vi "Skyline Send Waveform File.vi"(8 "error in":errorcluster, 9 "properties":cluster{"Key":string, "Value":string}[](array[cluster]) caption="properties (null)", 11 "data in":waveform(dbl)[](array[waveform])) -> (0 "error out":errorcluster, 2 "size in bytes":i32, 3 "data out":waveform(dbl)[](array[waveform]))   [LabVIEW 2017, in "Logger.lvclass"]
uses:
  logger/Logger.lvclass
  <vilib>/Skyline/File/File/Send Buffer.vi
  <vilib>/Skyline/File/File/NI Skyline File.lvclass
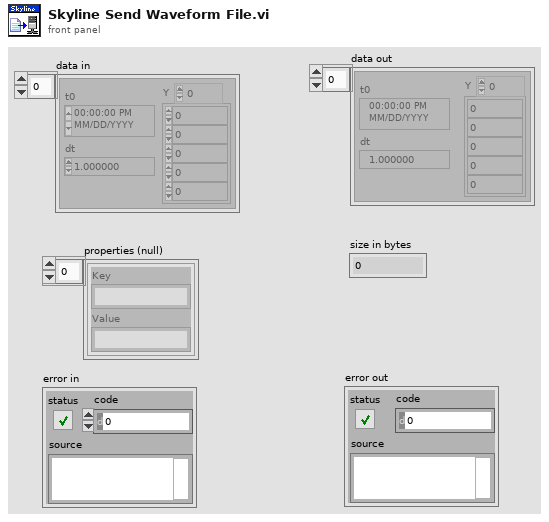
[diagram p1: front panel]
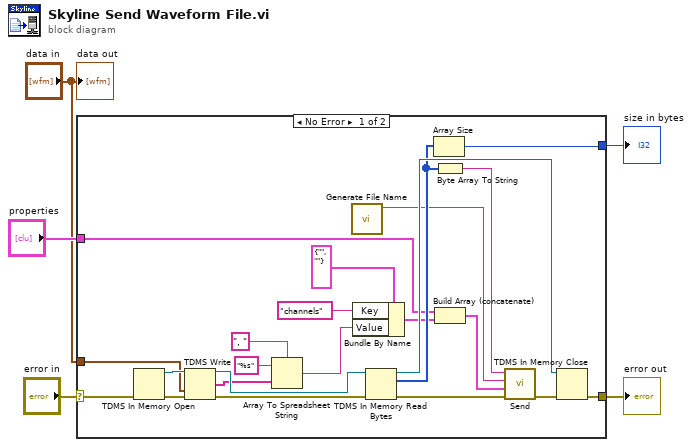
[diagram p0: block diagram]
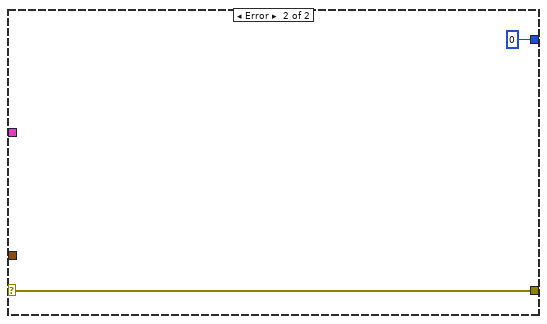
[diagram p2: hidden frame]
diagram:
  n1 = case shown="No Error" "error in" {
    selector: "error in" -> [w22 w30]
    tunnel: [w24 w30] -> w5
    tunnel: "properties" -> [w12 _]
    tunnel: "data in" -> [w27 _]
    tunnel: [w20 0] -> w1
    frame No Error {
      n2 = TDMS In Memory Open(8:w22) -> (0:w23:errorcluster, 3:w28:refnum<k34>)  [unwired: 1 in]
      n3 = TDMS Write(0:w28, 9:w27, 11:w23) -> (4:w19:refnum<k34>, 8:w17:string[], 15:w26:errorcluster)  [unwired: 3 in, 1 out]
      n4 = Array To Spreadsheet String(delimiter (Tab)=", ", array=w17, 3:"%s" ("format string")) -> (spreadsheet string=w13:string)
      n5 = call "Generate File Name.vi"() -> ("file name"=w10:string)  [unwired: 11 in]
      n6 = Bundle By Name(cluster=cluster{"Key":string, "Value":string} {"Key"="", "Value"=""} ("Property"), "Key"="channels", "Value"=w13) -> (w11:cluster{"Key":string, "Value":string})
      n7 = TDMS In Memory Read Bytes(8:w26, 11:w19) -> (0:w7:errorcluster, 2:w21:u8[], 3:w25:refnum<k34>)  [unwired: 2 in]
      n8 = Array Size(array=w21) -> (size(s)=w20:i32)
      n9 = Byte Array To String(unsigned byte array=w21) -> (string=w9:string)
      n10 = Build Array (concatenate)(w12, w11) -> (w8:cluster{"Key":string, "Value":string}[])
      n11 = call-poly <vilib>:"Send.vi"("error in (no error)"=w7, "properties"=w8, "file name"=w10, "data"=w9) -> ("error out"=w6:errorcluster)  [unwired: 5 in, 1 out]
      n12 = TDMS In Memory Close(8:w6, 11:w25) -> (0:w24:errorcluster)  [unwired: 2 in]
    }
    frame Error {
    }
  }
  "error out" <- w5
  "size in bytes" <- w1
  "data out" <- "data in"
